vi "Single Slow IV v1.1.vi"() -> ()   [LabVIEW 2018]
uses:
  <vilib>/Utility/file.llb/Write Delimited Spreadsheet (DBL).vi
panel:
  in  "stop":bool
  in  "Tab Control 2":enum32{"Plot 0", "Plot 1", "Plot 2", "Plot 3"}(tab)
  out "I vs Chan 0":cluster{"Y":dbl[], "Y":dbl[]}[](graph)=[{"Y"=[-10.0, -9.9, -9.8, -9.7, -9.6, -9.5, -9.399999999999999, -9.299999999999999, -9.200000000000001, -9.1, -9.0, -8.9, -8.8, -8.7, -8.6, -8.5, -8.4, -8.299999999999999, -8.200000000000001, -8.100000000000001, -8.0, -7.9, -7.800000000000001, -7.7, -7.6, -7.5, -7.4, -7.3, -7.199999999999999, -7.1, -7.0, -6.8999999999999995, -6.799999999999999, -6.699999999999999, -6.6, -6.499999999999999, -6.4, -6.3, -6.2, -6.1, -6.0, -5.8999999999999995, -5.800000000000001, -5.700000000000001, -5.6000000000000005, -5.5, -5.4, -5.300000000000001, -5.2, -5.1, -5.0, -4.9, -4.8, -4.699999999999999, -4.6, -4.5, -4.3999999999999995, -4.299999999999999, -4.2, -4.1000000000000005, -4.0, -3.9000000000000004, -3.8, -3.7, -3.5999999999999996, -3.5, -3.3999999999999995, -3.3, -3.1999999999999993, -3.0999999999999996, -2.999999999999999, -2.9000000000000004, -2.8000000000000003, -2.7, -2.6, -2.5, -2.4, -2.3, -2.1999999999999997, -2.0999999999999996, -1.9999999999999996, -1.8999999999999995, -1.7999999999999994, -1.6999999999999993, -1.6000000000000003, -1.5000000000000002, -1.4000000000000001, -1.3, -1.2, -1.0999999999999999, -0.9999999999999998, -0.8999999999999997, -0.7999999999999996, -0.6999999999999995, -0.5999999999999994, -0.49999999999999933, -0.40000000000000036, -0.30000000000000027, -0.20000000000000018, -0.10000000000000009, 0.0, 0.10000000000000009, 0.20000000000000018, 0.30000000000000027, 0.40000000000000036, 0.5000000000000004, 0.6000000000000005, 0.7000000000000006, 0.8000000000000007, 0.9000000000000008, 1.0000000000000009, 1.100000000000001, 1.200000000000001, 1.3000000000000012, 1.4000000000000012, 1.5000000000000013, 1.5999999999999992, 1.6999999999999993, 1.7999999999999994, 1.8999999999999995, 1.9999999999999996, 2.0999999999999996, 2.1999999999999997, 2.3, 2.4, 2.5, 2.6, 2.7, 2.8000000000000003, 2.9000000000000004, 3.0000000000000004, 3.1000000000000005, 3.2000000000000006, 3.3000000000000007, 3.400000000000001, 3.500000000000001, 3.600000000000001, 3.700000000000001, 3.800000000000001, 3.9000000000000012, 4.000000000000002, 4.1, 4.199999999999999, 4.299999999999999, 4.3999999999999995, 4.5, 4.6, 4.699999999999999, 4.8, 4.9, 5.0, 5.1, 5.2, 5.300000000000001, 5.4, 5.5, 5.6000000000000005, 5.700000000000001, 5.800000000000001, 5.9, 6.000000000000001, 6.100000000000001, 6.200000000000001, 6.300000000000001, 6.400000000000001, 6.500000000000002, 6.600000000000001, 6.699999999999999, 6.799999999999999, 6.8999999999999995, 7.0, 7.1, 7.199999999999999, 7.3, 7.4, 7.5, 7.6, 7.7, 7.800000000000001, 7.9, 8.0, 8.100000000000001, 8.200000000000001, 8.3, 8.4, 8.5, 8.600000000000001, 8.700000000000001, 8.8, 8.900000000000002, 9.000000000000002, 9.100000000000001, 9.2, 9.299999999999999, 9.399999999999999, 9.5, 9.6, 9.7, 9.8, 9.9, 10.0], "Y"=[-0.00012308349609375, -0.0001234375, -0.00012093505859375, -0.00011771240234374999, -0.00011741943359375, -0.0001174072265625, -0.00011278076171874999, -0.00011287841796875001, -0.000112548828125, -0.00011116943359375001, -0.00010870361328125001, -0.00010834960937500001, -0.00010524902343750001, -0.00010374755859375, -0.00010172119140624999, -0.000101708984375, -0.00010029296875, -9.809570312500001e-05, -9.749755859375001e-05, -9.554443359375001e-05, -9.404296875e-05, -9.383544921875e-05, -9.218750000000001e-05, -8.903808593749999e-05, -8.939208984375e-05, -8.759765625e-05, -8.40087890625e-05, -8.4423828125e-05, -8.291015625e-05, -8.004150390625001e-05, -7.958984375e-05, -7.987060546875e-05, -7.769775390625001e-05, -7.576904296875e-05, -7.4658203125e-05, -7.2802734375e-05, -7.19482421875e-05, -7.186279296875001e-05, -6.826171875e-05, -6.763916015625e-05, -6.571044921875e-05, -6.614990234374999e-05, -6.256103515625e-05, -6.253662109375e-05, -5.97900390625e-05, -6.002197265625e-05, -5.882568359375e-05, -5.814208984375e-05, -5.416259765625e-05, -5.549316406250001e-05, -5.067138671875e-05, -5.35888671875e-05, -5.003662109375e-05, -4.7900390624999996e-05, -4.786376953125e-05, -4.3701171875e-05, -4.373779296875e-05, -4.140625e-05, -4.14306640625e-05, -3.7939453125e-05, -3.98193359375e-05, -3.8134765625e-05, -3.443603515625e-05, -3.5791015625e-05, -3.282470703125e-05, -3.2153320312499996e-05, -2.8991699218750002e-05, -2.92724609375e-05, -2.63916015625e-05, -2.52197265625e-05, -2.432861328125e-05, -2.05810546875e-05, -2.22412109375e-05, -2.122802734375e-05, -1.9128417968749997e-05, -1.689453125e-05, -1.826171875e-05, -1.612548828125e-05, -1.339111328125e-05, -1.2646484375e-05, -1.1462402343750001e-05, -9.99755859375e-06, -1.046142578125e-05, -8.5205078125e-06, -5.3466796875e-06, -4.101562500000001e-06, -5.944824218750001e-06, -2.099609375e-06, -1.2695312500000002e-06, 2.3193359375e-07, 3.18603515625e-06, 3.3691406250000004e-06, 6.4941406250000005e-06, 6.99462890625e-06, 6.99462890625e-06, 9.66796875e-06, 1.053466796875e-05, 1.2292480468750001e-05, 1.484375e-05, 1.5002441406250001e-05, 1.539306640625e-05, 1.497802734375e-05, 1.7041015625e-05, 2.073974609375e-05, 1.790771484375e-05, 1.9860839843749998e-05, 2.314453125e-05, 2.535400390625e-05, 2.801513671875e-05, 3.09814453125e-05, 2.987060546875e-05, 3.109130859375e-05, 3.3544921875000005e-05, 3.33984375e-05, 3.372802734375e-05, 3.5546875e-05, 3.8281250000000006e-05, 3.77685546875e-05, 3.85986328125e-05, 4.088134765625e-05, 4.32373046875e-05, 4.583740234375e-05, 4.6875e-05, 4.798583984375e-05, 4.942626953125e-05, 4.9621582031250003e-05, 4.8864746093750005e-05, 5.260009765625e-05, 5.27587890625e-05, 5.6555175781250006e-05, 5.62255859375e-05, 5.919189453125e-05, 5.92529296875e-05, 5.968017578125e-05, 6.07666015625e-05, 6.392822265625e-05, 6.356201171875e-05, 6.614990234374999e-05, 6.651611328124999e-05, 7.0654296875e-05, 6.744384765625e-05, 7.159423828125e-05, 7.252197265625001e-05, 7.586669921875e-05, 7.644042968750001e-05, 8.035888671875e-05, 7.917480468750001e-05, 8.00048828125e-05, 8.186035156250001e-05, 8.016357421875001e-05, 8.482666015625e-05, 8.565673828125001e-05, 8.717041015625001e-05, 8.928222656249999e-05, 8.980712890625e-05, 9.084472656250001e-05, 9.117431640625e-05, 9.261474609375e-05, 9.58251953125e-05, 9.794921875e-05, 9.8876953125e-05, 0.0001031494140625, 0.00010015869140625, 0.00010286865234375001, 0.00010465087890625, 0.00010682373046875, 0.00010622558593750001, 0.00011091308593750001, 0.00011068115234375001, 0.00010891113281250001, 0.000113916015625, 0.00011505126953125, 0.00011524658203125, 0.00011818847656250001, 0.00011900634765625, 0.00012003173828125, 0.00012119140625, 0.0001236083984375, 0.000122900390625, 0.0001267822265625, 0.00012701416015625, 0.00012807617187500002, 0.00013043212890625, 0.00013155517578125, 0.00013193359375, 0.00013393554687500002, 0.00013890380859375002, 0.00013798828125, 0.00013800048828125, 0.00014044189453125, 0.00014061279296875002, 0.000144677734375, 0.0001461181640625, 0.000145361328125, 0.00014764404296875, 0.00014439697265625, 0.00014951171874999999, 0.00014968261718750002, 0.00015272216796874999, 0.00015264892578125, 0.000153466796875]}]
  out "Name 0":string="DC Voltage V"
  out "I vs Chan 1":cluster{"Y":dbl[], "Y":dbl[]}[](graph)=[{"Y"=[-10.0, -9.9, -9.8, -9.7, -9.6, -9.5, -9.399999999999999, -9.299999999999999, -9.200000000000001, -9.1, -9.0, -8.9, -8.8, -8.7, -8.6, -8.5, -8.4, -8.299999999999999, -8.200000000000001, -8.100000000000001, -8.0, -7.9, -7.800000000000001, -7.7, -7.6, -7.5, -7.4, -7.3, -7.199999999999999, -7.1, -7.0, -6.8999999999999995, -6.799999999999999, -6.699999999999999, -6.6, -6.499999999999999, -6.4, -6.3, -6.2, -6.1, -6.0, -5.8999999999999995, -5.800000000000001, -5.700000000000001, -5.6000000000000005, -5.5, -5.4, -5.300000000000001, -5.2, -5.1, -5.0, -4.9, -4.8, -4.699999999999999, -4.6, -4.5, -4.3999999999999995, -4.299999999999999, -4.2, -4.1000000000000005, -4.0, -3.9000000000000004, -3.8, -3.7, -3.5999999999999996, -3.5, -3.3999999999999995, -3.3, -3.1999999999999993, -3.0999999999999996, -2.999999999999999, -2.9000000000000004, -2.8000000000000003, -2.7, -2.6, -2.5, -2.4, -2.3, -2.1999999999999997, -2.0999999999999996, -1.9999999999999996, -1.8999999999999995, -1.7999999999999994, -1.6999999999999993, -1.6000000000000003, -1.5000000000000002, -1.4000000000000001, -1.3, -1.2, -1.0999999999999999, -0.9999999999999998, -0.8999999999999997, -0.7999999999999996, -0.6999999999999995, -0.5999999999999994, -0.49999999999999933, -0.40000000000000036, -0.30000000000000027, -0.20000000000000018, -0.10000000000000009, 0.0, 0.10000000000000009, 0.20000000000000018, 0.30000000000000027, 0.40000000000000036, 0.5000000000000004, 0.6000000000000005, 0.7000000000000006, 0.8000000000000007, 0.9000000000000008, 1.0000000000000009, 1.100000000000001, 1.200000000000001, 1.3000000000000012, 1.4000000000000012, 1.5000000000000013, 1.5999999999999992, 1.6999999999999993, 1.7999999999999994, 1.8999999999999995, 1.9999999999999996, 2.0999999999999996, 2.1999999999999997, 2.3, 2.4, 2.5, 2.6, 2.7, 2.8000000000000003, 2.9000000000000004, 3.0000000000000004, 3.1000000000000005, 3.2000000000000006, 3.3000000000000007, 3.400000000000001, 3.500000000000001, 3.600000000000001, 3.700000000000001, 3.800000000000001, 3.9000000000000012, 4.000000000000002, 4.1, 4.199999999999999, 4.299999999999999, 4.3999999999999995, 4.5, 4.6, 4.699999999999999, 4.8, 4.9, 5.0, 5.1, 5.2, 5.300000000000001, 5.4, 5.5, 5.6000000000000005, 5.700000000000001, 5.800000000000001, 5.9, 6.000000000000001, 6.100000000000001, 6.200000000000001, 6.300000000000001, 6.400000000000001, 6.500000000000002, 6.600000000000001, 6.699999999999999, 6.799999999999999, 6.8999999999999995, 7.0, 7.1, 7.199999999999999, 7.3, 7.4, 7.5, 7.6, 7.7, 7.800000000000001, 7.9, 8.0, 8.100000000000001, 8.200000000000001, 8.3, 8.4, 8.5, 8.600000000000001, 8.700000000000001, 8.8, 8.900000000000002, 9.000000000000002, 9.100000000000001, 9.2, 9.299999999999999, 9.399999999999999, 9.5, 9.6, 9.7, 9.8, 9.9, 10.0], "Y"=[-9.593505859375, -9.5345458984375, -9.409423828125, -9.3255615234375, -9.232177734375, -9.154541015625, -9.0064697265625, -8.9058837890625, -8.836181640625, -8.7589111328125, -8.6331787109375, -8.5640869140625, -8.447265625, -8.3675537109375, -8.2216796875, -8.175537109375, -8.065185546875, -7.9620361328125, -7.8717041015625, -7.77880859375, -7.6875, -7.6253662109375, -7.516357421875, -7.3792724609375, -7.2818603515625, -7.2069091796875, -7.0982666015625, -7.0257568359375, -6.923583984375, -6.798583984375, -6.7196044921875, -6.6395263671875, -6.5299072265625, -6.4405517578125, -6.3487548828125, -6.248046875, -6.1641845703125, -6.0799560546875, -5.965087890625, -5.882080078125, -5.7880859375, -5.7003173828125, -5.58544921875, -5.485595703125, -5.3775634765625, -5.3094482421875, -5.2239990234375, -5.120361328125, -4.9964599609375, -4.9444580078125, -4.79248046875, -4.744873046875, -4.6241455078125, -4.5133056640625, -4.4425048828125, -4.3153076171875, -4.248046875, -4.1307373046875, -4.0538330078125, -3.9373779296875, -3.8994140625, -3.782470703125, -3.6390380859375, -3.598388671875, -3.4920654296875, -3.395751953125, -3.2786865234375, -3.2120361328125, -3.0963134765625, -3.002197265625, -2.9107666015625, -2.75732421875, -2.713623046875, -2.621826171875, -2.535888671875, -2.4136962890625, -2.372802734375, -2.2467041015625, -2.124267578125, -2.048095703125, -1.9478759765625, -1.8392333984375, -1.8209228515625, -1.7073974609375, -1.562255859375, -1.4957275390625, -1.4473876953125, -1.306640625, -1.2362060546875, -1.1260986328125, -0.9921875, -0.931640625, -0.8140869140625, -0.73583984375, -0.6666259765625, -0.527587890625, -0.4603271484375, -0.361083984375, -0.2269287109375, -0.1763916015625, -0.08984375, 0.015380859375, 0.1270751953125, 0.263427734375, 0.3182373046875, 0.38037109375, 0.48974609375, 0.59765625, 0.70166015625, 0.8580322265625, 0.88330078125, 0.9742431640625, 1.094482421875, 1.1697998046875, 1.2156982421875, 1.35595703125, 1.4716796875, 1.5325927734375, 1.6243896484375, 1.7108154296875, 1.84130859375, 1.951171875, 2.045654296875, 2.146728515625, 2.2236328125, 2.3109130859375, 2.37353515625, 2.49951171875, 2.59033203125, 2.6856689453125, 2.7845458984375, 2.8961181640625, 2.9559326171875, 3.0474853515625, 3.1373291015625, 3.2685546875, 3.3409423828125, 3.439697265625, 3.530029296875, 3.6690673828125, 3.70556640625, 3.832275390625, 3.9168701171875, 4.0284423828125, 4.1300048828125, 4.2607421875, 4.3009033203125, 4.4122314453125, 4.49609375, 4.56201171875, 4.6815185546875, 4.7872314453125, 4.8818359375, 4.9942626953125, 5.055419921875, 5.160888671875, 5.231689453125, 5.3519287109375, 5.4739990234375, 5.56298828125, 5.6533203125, 5.7923583984375, 5.806396484375, 5.936767578125, 6.0274658203125, 6.14111328125, 6.2001953125, 6.37353515625, 6.431640625, 6.496826171875, 6.6165771484375, 6.7174072265625, 6.79345703125, 6.9200439453125, 6.97900390625, 7.0965576171875, 7.176025390625, 7.3065185546875, 7.365966796875, 7.5006103515625, 7.5654296875, 7.6612548828125, 7.7730712890625, 7.868408203125, 7.9364013671875, 8.0616455078125, 8.1871337890625, 8.2489013671875, 8.3131103515625, 8.435791015625, 8.5284423828125, 8.630126953125, 8.75, 8.8126220703125, 8.908203125, 8.9510498046875, 9.1063232421875, 9.17236328125, 9.272705078125, 9.370361328125, 9.4595947265625]}]
  out "Name 1":string="DC current uA"
  out "I vs Chan 2":cluster{"Y":dbl[], "Y":dbl[]}[](graph)=[{"Y"=[-10.0, -9.9, -9.8, -9.7, -9.6, -9.5, -9.399999999999999, -9.299999999999999, -9.200000000000001, -9.1, -9.0, -8.9, -8.8, -8.7, -8.6, -8.5, -8.4, -8.299999999999999, -8.200000000000001, -8.100000000000001, -8.0, -7.9, -7.800000000000001, -7.7, -7.6, -7.5, -7.4, -7.3, -7.199999999999999, -7.1, -7.0, -6.8999999999999995, -6.799999999999999, -6.699999999999999, -6.6, -6.499999999999999, -6.4, -6.3, -6.2, -6.1, -6.0, -5.8999999999999995, -5.800000000000001, -5.700000000000001, -5.6000000000000005, -5.5, -5.4, -5.300000000000001, -5.2, -5.1, -5.0, -4.9, -4.8, -4.699999999999999, -4.6, -4.5, -4.3999999999999995, -4.299999999999999, -4.2, -4.1000000000000005, -4.0, -3.9000000000000004, -3.8, -3.7, -3.5999999999999996, -3.5, -3.3999999999999995, -3.3, -3.1999999999999993, -3.0999999999999996, -2.999999999999999, -2.9000000000000004, -2.8000000000000003, -2.7, -2.6, -2.5, -2.4, -2.3, -2.1999999999999997, -2.0999999999999996, -1.9999999999999996, -1.8999999999999995, -1.7999999999999994, -1.6999999999999993, -1.6000000000000003, -1.5000000000000002, -1.4000000000000001, -1.3, -1.2, -1.0999999999999999, -0.9999999999999998, -0.8999999999999997, -0.7999999999999996, -0.6999999999999995, -0.5999999999999994, -0.49999999999999933, -0.40000000000000036, -0.30000000000000027, -0.20000000000000018, -0.10000000000000009, 0.0, 0.10000000000000009, 0.20000000000000018, 0.30000000000000027, 0.40000000000000036, 0.5000000000000004, 0.6000000000000005, 0.7000000000000006, 0.8000000000000007, 0.9000000000000008, 1.0000000000000009, 1.100000000000001, 1.200000000000001, 1.3000000000000012, 1.4000000000000012, 1.5000000000000013, 1.5999999999999992, 1.6999999999999993, 1.7999999999999994, 1.8999999999999995, 1.9999999999999996, 2.0999999999999996, 2.1999999999999997, 2.3, 2.4, 2.5, 2.6, 2.7, 2.8000000000000003, 2.9000000000000004, 3.0000000000000004, 3.1000000000000005, 3.2000000000000006, 3.3000000000000007, 3.400000000000001, 3.500000000000001, 3.600000000000001, 3.700000000000001, 3.800000000000001, 3.9000000000000012, 4.000000000000002, 4.1, 4.199999999999999, 4.299999999999999, 4.3999999999999995, 4.5, 4.6, 4.699999999999999, 4.8, 4.9, 5.0, 5.1, 5.2, 5.300000000000001, 5.4, 5.5, 5.6000000000000005, 5.700000000000001, 5.800000000000001, 5.9, 6.000000000000001, 6.100000000000001, 6.200000000000001, 6.300000000000001, 6.400000000000001, 6.500000000000002, 6.600000000000001, 6.699999999999999, 6.799999999999999, 6.8999999999999995, 7.0, 7.1, 7.199999999999999, 7.3, 7.4, 7.5, 7.6, 7.7, 7.800000000000001, 7.9, 8.0, 8.100000000000001, 8.200000000000001, 8.3, 8.4, 8.5, 8.600000000000001, 8.700000000000001, 8.8, 8.900000000000002, 9.000000000000002, 9.100000000000001, 9.2, 9.299999999999999, 9.399999999999999, 9.5, 9.6, 9.7, 9.8, 9.9, 10.0], "Y"=[0.14237060546875, 0.14224853515625, 0.13931884765625, 0.13436279296875, 0.13089599609375, 0.1484130859375, 0.1311767578125, 0.12135009765625, 0.126171875, 0.11885986328125, 0.12998046875, 0.1361572265625, 0.137744140625, 0.13939208984375, 0.14383544921875, 0.13359375, 0.1277099609375, 0.13414306640625, 0.1346923828125, 0.13975830078125, 0.12977294921875, 0.1345458984375, 0.13109130859375, 0.14085693359375, 0.1389892578125, 0.12850341796875, 0.132080078125, 0.1217529296875, 0.119287109375, 0.121826171875, 0.13089599609375, 0.13604736328125, 0.13546142578125, 0.12481689453125, 0.133984375, 0.14044189453125, 0.143896484375, 0.138916015625, 0.1323486328125, 0.1269287109375, 0.1247314453125, 0.13338623046875, 0.1311767578125, 0.1350341796875, 0.1343505859375, 0.1373291015625, 0.1375244140625, 0.14576416015625, 0.14306640625, 0.143408203125, 0.1353759765625, 0.1471435546875, 0.139111328125, 0.13782958984375, 0.14586181640625, 0.14405517578125, 0.12735595703125, 0.12763671875, 0.14405517578125, 0.1427734375, 0.131298828125, 0.135302734375, 0.134326171875, 0.13094482421875, 0.12060546875, 0.12052001953125, 0.12391357421875, 0.13721923828125, 0.13489990234375, 0.1359619140625, 0.1348388671875, 0.13406982421875, 0.1313232421875, 0.1314453125, 0.13187255859375, 0.128076171875, 0.12703857421875, 0.135888671875, 0.12996826171875, 0.1257080078125, 0.1363037109375, 0.12720947265625, 0.124462890625, 0.13179931640625, 0.13096923828125, 0.13603515625, 0.13265380859375, 0.1372314453125, 0.14005126953125, 0.13939208984375, 0.1390380859375, 0.14755859375, 0.14853515625, 0.15540771484375, 0.14439697265625, 0.15701904296875, 0.15970458984375, 0.14603271484375, 0.11851806640625, 0.08155517578125, 0.0737548828125, 0.059033203125, 0.0862548828125, 0.107373046875, 0.14686279296875, 0.153271484375, 0.16593017578125, 0.16634521484375, 0.15345458984375, 0.154052734375, 0.14573974609375, 0.13909912109375, 0.1457275390625, 0.144091796875, 0.13836669921875, 0.12183837890625, 0.12923583984375, 0.13216552734375, 0.13109130859375, 0.12672119140625, 0.12862548828125, 0.138720703125, 0.13399658203125, 0.13165283203125, 0.14306640625, 0.131005859375, 0.12864990234375, 0.124072265625, 0.13448486328125, 0.1269775390625, 0.13427734375, 0.12752685546875, 0.1389892578125, 0.1315185546875, 0.11864013671875, 0.119140625, 0.12742919921875, 0.13262939453125, 0.13258056640625, 0.13468017578125, 0.139892578125, 0.1356201171875, 0.1286865234375, 0.11729736328125, 0.12257080078125, 0.11641845703125, 0.137060546875, 0.14832763671875, 0.1409423828125, 0.13443603515625, 0.1446044921875, 0.13297119140625, 0.13448486328125, 0.1262451171875, 0.127734375, 0.131103515625, 0.14002685546875, 0.12392578125, 0.12786865234375, 0.11773681640625, 0.12716064453125, 0.12587890625, 0.1200439453125, 0.13533935546875, 0.12574462890625, 0.1306640625, 0.14171142578125, 0.1371826171875, 0.13031005859375, 0.1381591796875, 0.12945556640625, 0.13642578125, 0.14312744140625, 0.13961181640625, 0.14447021484375, 0.13270263671875, 0.1308349609375, 0.136376953125, 0.1431396484375, 0.13074951171875, 0.12476806640625, 0.1382568359375, 0.1403076171875, 0.1392578125, 0.12987060546875, 0.13812255859375, 0.14114990234375, 0.142626953125, 0.1402587890625, 0.14439697265625, 0.145849609375, 0.14061279296875, 0.12906494140625, 0.1228759765625, 0.12764892578125, 0.130908203125, 0.134765625, 0.1360107421875, 0.13594970703125, 0.13138427734375, 0.134765625]}]
  out "Name 2":string="dV V"
  out "I vs Chan 3":cluster{"Y":dbl[], "Y":dbl[]}[](graph)=[{"Y"=[-10.0, -9.9, -9.8, -9.7, -9.6, -9.5, -9.399999999999999, -9.299999999999999, -9.200000000000001, -9.1, -9.0, -8.9, -8.8, -8.7, -8.6, -8.5, -8.4, -8.299999999999999, -8.200000000000001, -8.100000000000001, -8.0, -7.9, -7.800000000000001, -7.7, -7.6, -7.5, -7.4, -7.3, -7.199999999999999, -7.1, -7.0, -6.8999999999999995, -6.799999999999999, -6.699999999999999, -6.6, -6.499999999999999, -6.4, -6.3, -6.2, -6.1, -6.0, -5.8999999999999995, -5.800000000000001, -5.700000000000001, -5.6000000000000005, -5.5, -5.4, -5.300000000000001, -5.2, -5.1, -5.0, -4.9, -4.8, -4.699999999999999, -4.6, -4.5, -4.3999999999999995, -4.299999999999999, -4.2, -4.1000000000000005, -4.0, -3.9000000000000004, -3.8, -3.7, -3.5999999999999996, -3.5, -3.3999999999999995, -3.3, -3.1999999999999993, -3.0999999999999996, -2.999999999999999, -2.9000000000000004, -2.8000000000000003, -2.7, -2.6, -2.5, -2.4, -2.3, -2.1999999999999997, -2.0999999999999996, -1.9999999999999996, -1.8999999999999995, -1.7999999999999994, -1.6999999999999993, -1.6000000000000003, -1.5000000000000002, -1.4000000000000001, -1.3, -1.2, -1.0999999999999999, -0.9999999999999998, -0.8999999999999997, -0.7999999999999996, -0.6999999999999995, -0.5999999999999994, -0.49999999999999933, -0.40000000000000036, -0.30000000000000027, -0.20000000000000018, -0.10000000000000009, 0.0, 0.10000000000000009, 0.20000000000000018, 0.30000000000000027, 0.40000000000000036, 0.5000000000000004, 0.6000000000000005, 0.7000000000000006, 0.8000000000000007, 0.9000000000000008, 1.0000000000000009, 1.100000000000001, 1.200000000000001, 1.3000000000000012, 1.4000000000000012, 1.5000000000000013, 1.5999999999999992, 1.6999999999999993, 1.7999999999999994, 1.8999999999999995, 1.9999999999999996, 2.0999999999999996, 2.1999999999999997, 2.3, 2.4, 2.5, 2.6, 2.7, 2.8000000000000003, 2.9000000000000004, 3.0000000000000004, 3.1000000000000005, 3.2000000000000006, 3.3000000000000007, 3.400000000000001, 3.500000000000001, 3.600000000000001, 3.700000000000001, 3.800000000000001, 3.9000000000000012, 4.000000000000002, 4.1, 4.199999999999999, 4.299999999999999, 4.3999999999999995, 4.5, 4.6, 4.699999999999999, 4.8, 4.9, 5.0, 5.1, 5.2, 5.300000000000001, 5.4, 5.5, 5.6000000000000005, 5.700000000000001, 5.800000000000001, 5.9, 6.000000000000001, 6.100000000000001, 6.200000000000001, 6.300000000000001, 6.400000000000001, 6.500000000000002, 6.600000000000001, 6.699999999999999, 6.799999999999999, 6.8999999999999995, 7.0, 7.1, 7.199999999999999, 7.3, 7.4, 7.5, 7.6, 7.7, 7.800000000000001, 7.9, 8.0, 8.100000000000001, 8.200000000000001, 8.3, 8.4, 8.5, 8.600000000000001, 8.700000000000001, 8.8, 8.900000000000002, 9.000000000000002, 9.100000000000001, 9.2, 9.299999999999999, 9.399999999999999, 9.5, 9.6, 9.7, 9.8, 9.9, 10.0], "Y"=[0.94891357421875, 0.9578369140625, 0.94735107421875, 0.9477783203125, 0.94619140625, 0.95455322265625, 0.95579833984375, 0.94427490234375, 0.9491455078125, 0.9447021484375, 0.94097900390625, 0.9394775390625, 0.95335693359375, 0.9498779296875, 0.94693603515625, 0.9442138671875, 0.949609375, 0.947998046875, 0.952978515625, 0.9468017578125, 0.95482177734375, 0.9583984375, 0.947021484375, 0.94285888671875, 0.9375, 0.940478515625, 0.9356689453125, 0.94532470703125, 0.9408447265625, 0.93841552734375, 0.94471435546875, 0.93890380859375, 0.95328369140625, 0.93822021484375, 0.9506591796875, 0.94007568359375, 0.950927734375, 0.9435546875, 0.95013427734375, 0.9459716796875, 0.950537109375, 0.95440673828125, 0.95286865234375, 0.9526611328125, 0.95450439453125, 0.95272216796875, 0.95611572265625, 0.950537109375, 0.955322265625, 0.9569091796875, 0.957177734375, 0.93946533203125, 0.95079345703125, 0.952880859375, 0.9504150390625, 0.9560302734375, 0.94222412109375, 0.9494140625, 0.956005859375, 0.9582275390625, 0.95799560546875, 0.94637451171875, 0.9373046875, 0.94144287109375, 0.95390625, 0.94190673828125, 0.9397216796875, 0.9546142578125, 0.94547119140625, 0.9369384765625, 0.95045166015625, 0.94356689453125, 0.942578125, 0.94906005859375, 0.9567626953125, 0.943408203125, 0.94183349609375, 0.95521240234375, 0.9445068359375, 0.95048828125, 0.9523681640625, 0.95489501953125, 0.95279541015625, 0.9577880859375, 0.95416259765625, 0.95416259765625, 0.9467529296875, 0.94588623046875, 0.94029541015625, 0.9417236328125, 0.954345703125, 0.954736328125, 0.94490966796875, 0.94364013671875, 0.93758544921875, 0.95206298828125, 0.954296875, 0.94566650390625, 0.9493408203125, 0.95355224609375, 0.9425537109375, 0.94534912109375, 0.9372314453125, 0.93629150390625, 0.93914794921875, 0.9525146484375, 0.94290771484375, 0.94998779296875, 0.95157470703125, 0.94967041015625, 0.94981689453125, 0.94427490234375, 0.95389404296875, 0.94150390625, 0.94864501953125, 0.94586181640625, 0.951708984375, 0.9447021484375, 0.94300537109375, 0.9546142578125, 0.95369873046875, 0.95408935546875, 0.94371337890625, 0.945654296875, 0.9428466796875, 0.95032958984375, 0.946044921875, 0.95467529296875, 0.9572998046875, 0.94462890625, 0.95084228515625, 0.949560546875, 0.94622802734375, 0.94490966796875, 0.94464111328125, 0.94300537109375, 0.94691162109375, 0.94111328125, 0.93807373046875, 0.94560546875, 0.946630859375, 0.9541015625, 0.9412353515625, 0.9434814453125, 0.95244140625, 0.95382080078125, 0.955419921875, 0.95010986328125, 0.94884033203125, 0.9486572265625, 0.94893798828125, 0.94495849609375, 0.9525146484375, 0.95382080078125, 0.9568359375, 0.944921875, 0.95164794921875, 0.9466064453125, 0.9466552734375, 0.94083251953125, 0.93809814453125, 0.93897705078125, 0.94224853515625, 0.9445068359375, 0.94974365234375, 0.9420166015625, 0.94814453125, 0.9400634765625, 0.9485107421875, 0.94620361328125, 0.947998046875, 0.94503173828125, 0.941162109375, 0.94833984375, 0.9508544921875, 0.9482177734375, 0.9396240234375, 0.9502685546875, 0.95997314453125, 0.96004638671875, 0.9498779296875, 0.94691162109375, 0.95335693359375, 0.95001220703125, 0.94827880859375, 0.943408203125, 0.9549560546875, 0.9496826171875, 0.9443603515625, 0.94561767578125, 0.94581298828125, 0.9424072265625, 0.95430908203125, 0.94036865234375, 0.9526611328125, 0.9468017578125, 0.954443359375, 0.94600830078125, 0.94906005859375, 0.9413330078125, 0.93865966796875]}]
  out "Name 3":string="dI uA"
  in  "Tab Control":T1(tab)
  in  "cRIO IP":string="//172.22.11.2"
  in  "Reading Average times":i32=20
  out "Unit":string
  in  "Tab Control 3":enum32{"Current", "Magnetic field"}(tab)
  in  "Delay Time s":dbl=0.15 caption="Delay Time (s)"
  in  "AO Channel":string(combo)="AO0"
  in  "current output Scale factor":dbl=10.0
  in  "Device Select":string(combo)="Elsa Magnet"
  in  "Fixed current uA":dbl
  in  "Scale factor":dbl
  in  "Field Rate mT per sec":dbl=0.1 format="%#_13g"
  in  "Start":dbl=-10.0
  in  "Current Range":dbl=20.0
  in  "Current Step":dbl=0.1
  in  "Ramp type":string(combo)="Range"
  in  "Ramp up first T":bool=TRUE
  in  "Channel name 0":string(combo)="DC Voltage V"
  in  "Scale factor0":dbl=0.001
  in  "Scale factor1":dbl=10.0
  in  "Channel name 1":string(combo)="DC current uA"
  in  "Chan 1":bool=TRUE
  in  "Scale factor2":dbl=1.0
  in  "Channel name 2":string(combo)="dV V"
  in  "Chan 2":bool=TRUE
  in  "Scale factor3":dbl=1.0
  in  "Channel name 3":string(combo)="dI uA"
  in  "Chan 3":bool=TRUE
  in  "Contour plot folder":path=path "C:/Users/gyue/Box/Guang Yue uiuc research box folder/data"
  out "error out":errorcluster
  # "Voltage x factor=uA"
  # "Voltage x factor=uA"
  # "Voltage x factor=actual"
  # "Voltage x factor=actual"
  # "Voltage x factor=actual"
  # "Voltage x factor=actual"
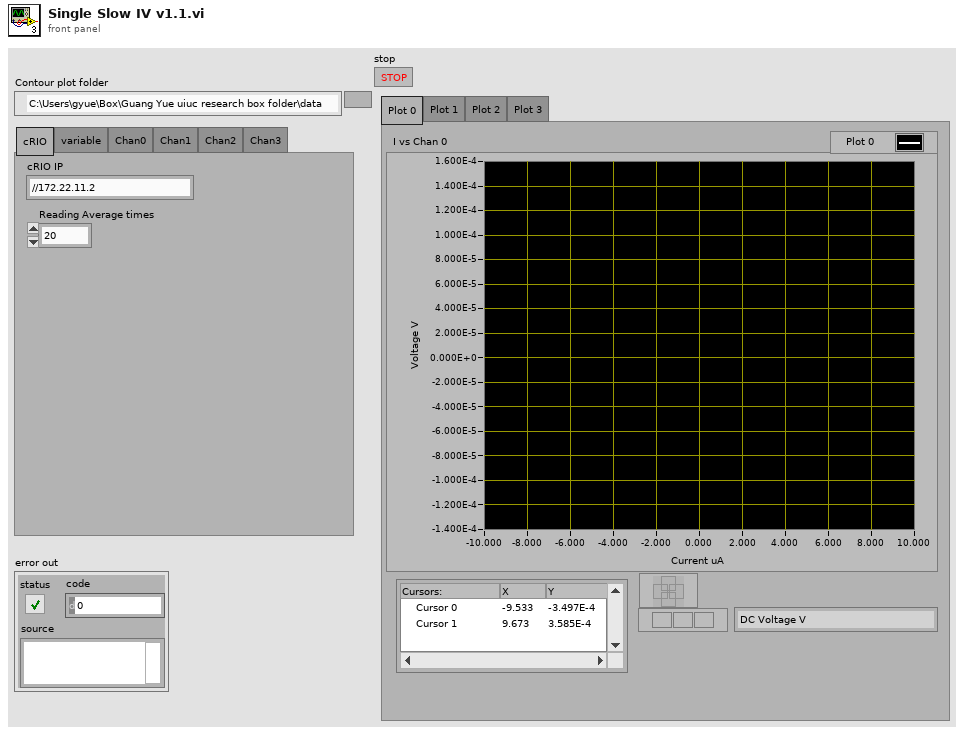
[diagram p1: front panel]
types:
  T1 = enum32{"cRIO", "variable", "Chan0", "Chan1", "Chan2", "Chan3"}
  T2 = cluster{"AI0":dbl, "AI1":dbl, "AI2":dbl, "AI3":dbl}
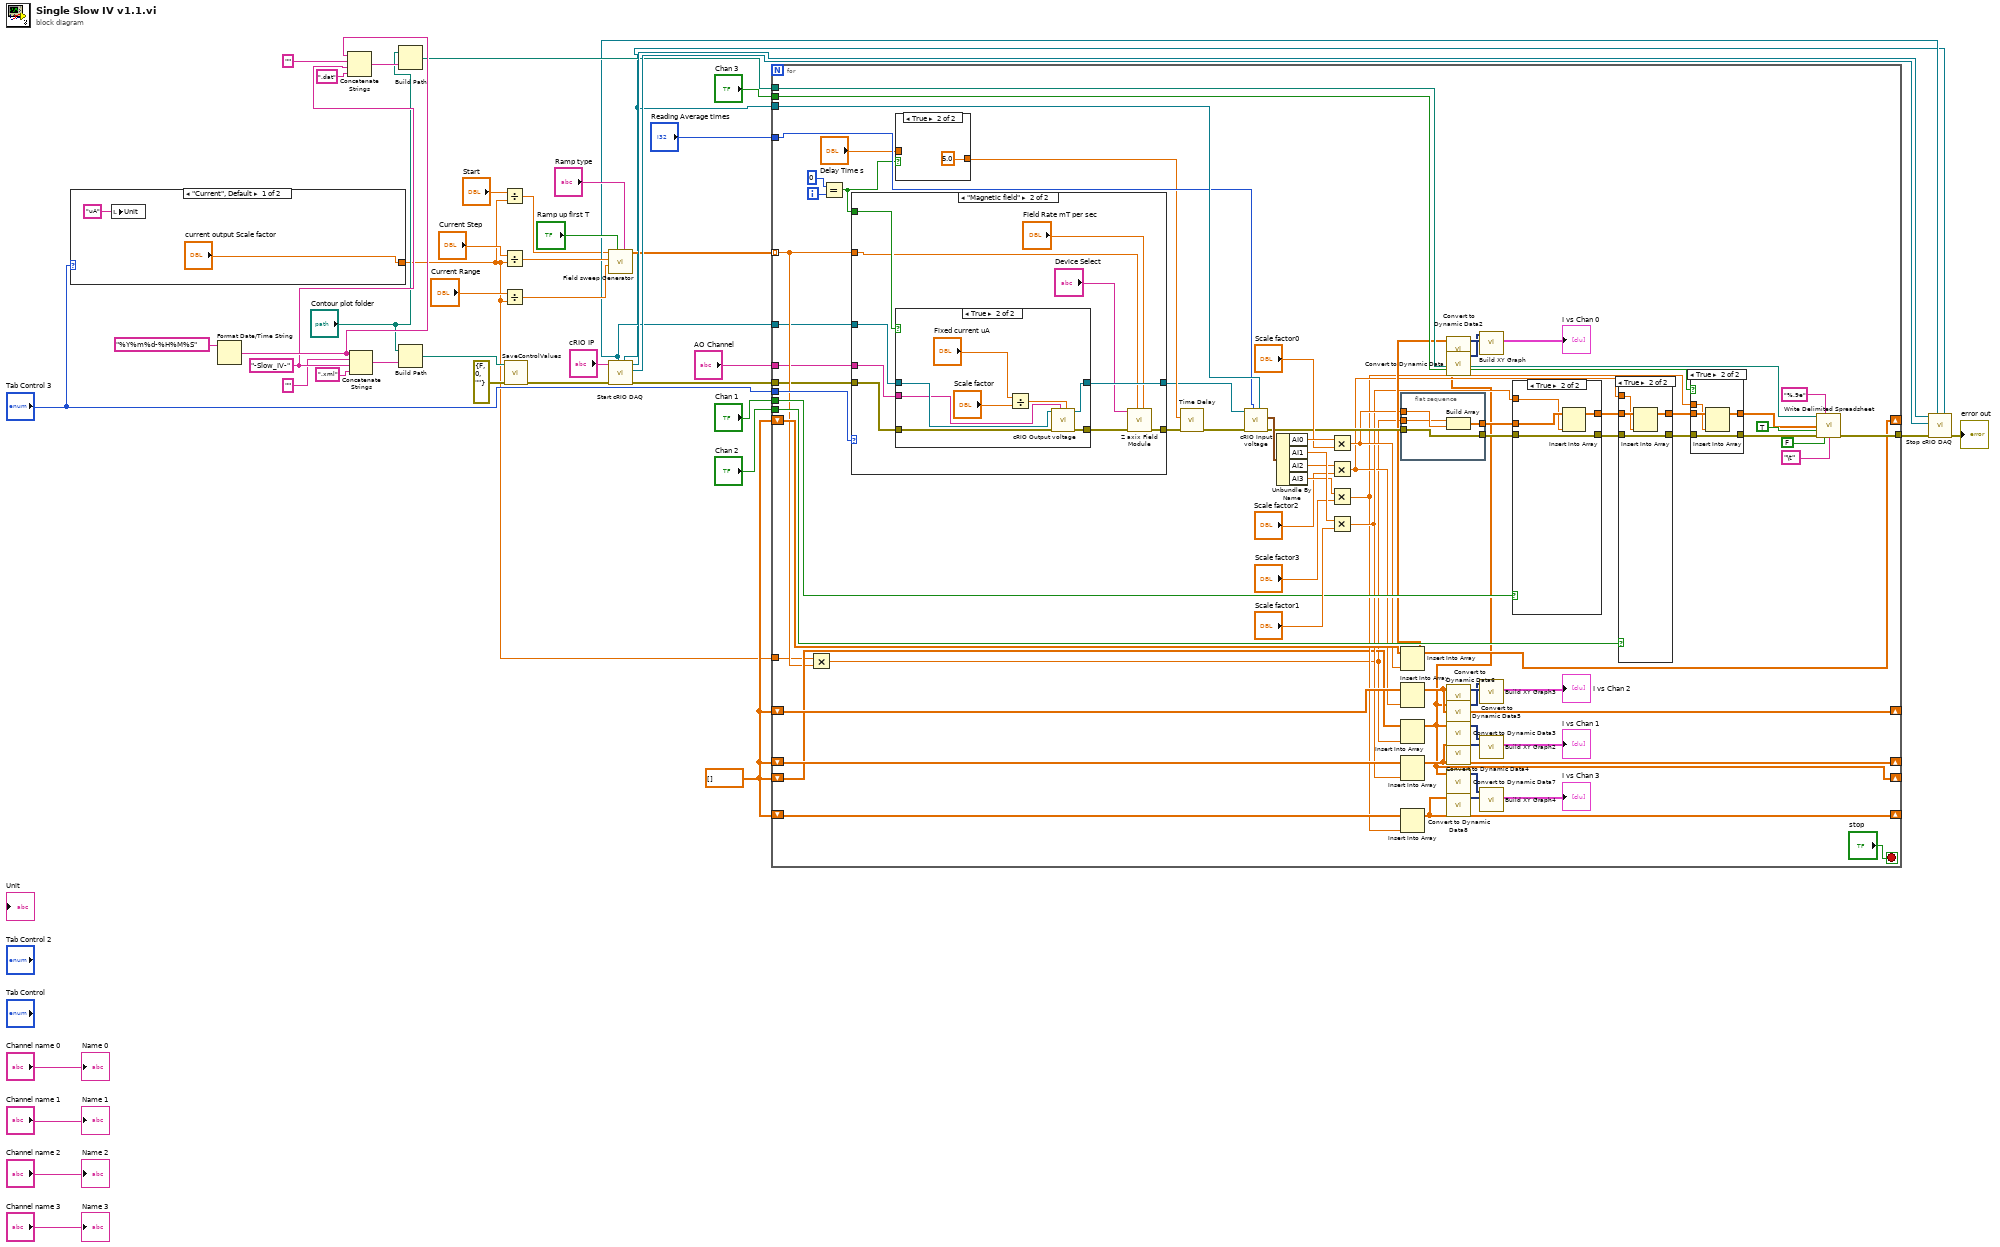
[diagram p0: block diagram]
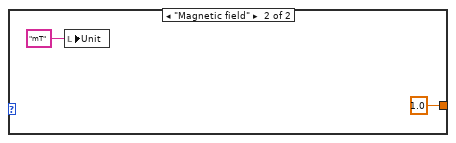
[diagram p2: hidden frame]
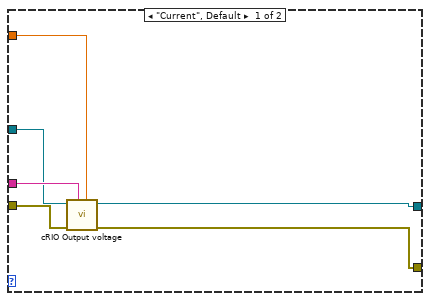
[diagram p3: hidden frame]
diagram:
  w11 = dbl[] []
  w36 = "-Slow_IV-"
  n1 = case shown="\"Current\", Default" "Tab Control 3" {
    tunnel: ["current output Scale factor" 1.0 ("current output Scale factor")] -> w1
    frame "Current", Default {
      n2 = local write "Unit"("uA" ("Unit")) -> ()
    }
    frame "Magnetic field" {
      n3 = local write "Unit"("mT" ("Unit")) -> ()
    }
  }
  n4 = Format Date/Time String(time format string (%c)="%Y%m%d-%H%M%S") -> (date/time string=w37:string)  [unwired: 2 in]
  n5 = Concatenate Strings(w37, "" ("string"), w36, ".dat" ("string")) -> (w39:string)
  n6 = Concatenate Strings(w37, "" ("string"), w36, ".xml" ("string")) -> (w42:string)
  n7 = Build Path(base path="Contour plot folder", name or relative path=w39) -> (appended path=w19:path)
  n8 = Build Path(base path="Contour plot folder", name or relative path=w42) -> (appended path=w40:path)
  n9 = Divide(x="Start", y=w1) -> (x/y=w3:dbl)
  n10 = Divide(x="Current Step", y=w1) -> (x/y=w24:dbl)
  n11 = Divide(x="Current Range", y=w1) -> (x/y=w23:dbl)
  n12 = call "SaveControlValues.vi"("XML File Path"=w40, "error in (no error)"=errorcluster {"status"=FALSE, "code"=0, "source"=""} ("error in")) -> ("error out"=w33:errorcluster)  [unwired: 8 in]
  n13 = call "Field sweep Generator.vi"("Ramp type"="Ramp type", "Ramp up first T"="Ramp up first T", "Field Radius"=w23, "Field step"=w24, "Field Origin"=w3) -> ("output array"=w20:dbl[])  [unwired: 6 in]
  n14 = call "Start cRIO DAQ.vi"("error in (no error)"=w33, "cRIO IP"="cRIO IP") -> ("error out"=w22:errorcluster, "vi reference"=w31:refnum<vi>, "application reference"=w32:refnum<vi>, "DAQ_AI_Reader endpoint"=w17:refnum<k21>, "DAQ_CMD_Writer endpoint"=w18:refnum<k21>)  [unwired: 5 in]
  n15 = for {
    tunnel: w22 -> [w53]
    tunnel: w18 -> [w52]
    tunnel: "AO Channel" -> [w54]
    tunnel: w20 -> [w55] mode=indexing
    tunnel: w17 -> [w118]
    tunnel: w19 -> [w117]
    tunnel: "Chan 1" -> [w99]
    tunnel: "Chan 2" -> [w98]
    tunnel: "Chan 3" -> [w97]
    tunnel: [w78] -> w10
    shift-right: [w73] -> _
    shift-left: w11 -> [w77]
    shift-right: [w72] -> _
    shift-left: w11 -> [w76]
    shift-right: [w71] -> _
    shift-left: w11 -> [w75]
    shift-right: [w70] -> _
    shift-left: w11 -> [w74]
    shift-right: [w63] -> _
    shift-left: w11 -> [w65]
    tunnel: "Reading Average times" -> [w62]
    tunnel: "Tab Control 3" -> [w56]
    tunnel: w1 -> [w48]
    i -> [w60]
    stop <- "stop" stop-if-true
    n16 = Multiply(x=w48, y=w55) -> (x*y=w64:dbl)
    n17 = Equal?(x=0, y=w60) -> (x = y?=w49:bool)
    n18 = case shown="\"Magnetic field\"" w56 {
      tunnel: w55 -> [w124 w125]
      tunnel: w54 -> [w123 w130]
      tunnel: w53 -> [w122 w133]
      tunnel: w52 -> [w121 w132]
      tunnel: [w120 w128] -> w51
      tunnel: [w119 w131] -> w50
      tunnel: w49 -> [_ w134]
      frame "Current", Default {
        n19 = call "cRIO Output voltage.vi"("Voltage"=w124, "AO Channel"=w123, "error in (no error)"=w122, "DAQ_CMD_Writer endpoint"=w121) -> ("error out"=w120:errorcluster, "DAQ_CMD_Writer endpoint out"=w119:refnum<k21>)  [unwired: 6 in]
      }
      frame "Magnetic field" {
        n20 = case shown="True" w134 {
          tunnel: w133 -> [w135 w144]
          tunnel: [w135 w143] -> w129
          tunnel: w132 -> [w136 w142]
          tunnel: [w136 w141] -> w131
          tunnel: w130 -> [_ w140]
          frame False {
          }
          frame True {
            n21 = Divide(x="Fixed current uA", y="Scale factor") -> (x/y=w138:dbl)
            n22 = call "cRIO Output voltage.vi"("Voltage"=w138, "AO Channel"=w140, "error in (no error)"=w144, "DAQ_CMD_Writer endpoint"=w142) -> ("error out"=w143:errorcluster, "DAQ_CMD_Writer endpoint out"=w141:refnum<k21>)  [unwired: 6 in]
          }
        }
        n23 = call "Z axix Field Module.vi"("Field Rate mT per sec"="Field Rate mT per sec", "Field Target mT"=w125, "error in (no error)"=w129, "Device Select"="Device Select") -> ("error out"=w128:errorcluster)  [unwired: 7 in]
      }
    }
    n24 = case shown="True" w49 {
      tunnel: "Delay Time s" -> [w145 _]
      tunnel: [w145 5.0 ("Delay Time s")] -> w57
      frame False {
      }
      frame True {
      }
    }
    n25 = call "Time Delay"("error in (no error)"=w51, "Delay Time (s)"=w57) -> ("error out"=w110:errorcluster)  [unwired: 9 in]
    n26 = call "cRIO Input voltage.vi"("DAQ_AI_Reader endpoint"=w118, "Average"=w62, "error in (no error)"=w110, "DAQ_CMD_Writer endpoint"=w50) -> ("error out"=w94:errorcluster, "output cluster"=w109:T2)  [unwired: 5 in, 1 out]
    n27 = Unbundle By Name(w109) -> ("AI0"=w108:dbl, "AI1"=w107:dbl, "AI2"=w106:dbl, "AI3"=w105:dbl)
    n28 = Multiply(x=w108, y="Scale factor0") -> (x*y=w69:dbl)
    n29 = Multiply(x=w106, y="Scale factor2") -> (x*y=w67:dbl)
    n30 = Multiply(x=w105, y="Scale factor3") -> (x*y=w66:dbl)
    n31 = Multiply(x=w107, y="Scale factor1") -> (x*y=w68:dbl)
    n32 = flat-sequence {
      tunnel: w94 -> [w150]
      tunnel: [w150] -> w93
      tunnel: w69 -> [w148]
      tunnel: [w149] -> w92
      tunnel: w64 -> [w147]
      frame #0 {
        n33 = Build Array(w147, w148) -> (w149:dbl[])
      }
    }
    n34 = Insert Into Array(array=w77, new element=w69) -> (w73:dbl[])  [unwired: 1 in]
    n35 = Insert Into Array(array=w75, new element=w67) -> (w71:dbl[])  [unwired: 1 in]
    n36 = Insert Into Array(array=w65, new element=w64) -> (w63:dbl[])  [unwired: 1 in]
    n37 = Insert Into Array(array=w76, new element=w68) -> (w72:dbl[])  [unwired: 1 in]
    n38 = Insert Into Array(array=w74, new element=w66) -> (w70:dbl[])  [unwired: 1 in]
    n39 = call "Convert to Dynamic Data2"("Array"=w73) -> ("Dynamic Data Type"=w113:dynamicdata)  [unwired: 3 in]
    n40 = call "Convert to Dynamic Data"("Array"=w63) -> ("Dynamic Data Type"=w112:dynamicdata)  [unwired: 3 in]
    n41 = call "Convert to Dynamic Data6"("Array"=w71) -> ("Dynamic Data Type"=w84:dynamicdata)  [unwired: 3 in]
    n42 = call "Convert to Dynamic Data5"("Array"=w63) -> ("Dynamic Data Type"=w83:dynamicdata)  [unwired: 3 in]
    n43 = call "Convert to Dynamic Data3"("Array"=w63) -> ("Dynamic Data Type"=w86:dynamicdata)  [unwired: 3 in]
    n44 = call "Convert to Dynamic Data4"("Array"=w72) -> ("Dynamic Data Type"=w87:dynamicdata)  [unwired: 3 in]
    n45 = call "Convert to Dynamic Data7"("Array"=w63) -> ("Dynamic Data Type"=w80:dynamicdata)  [unwired: 3 in]
    n46 = call "Convert to Dynamic Data8"("Array"=w70) -> ("Dynamic Data Type"=w81:dynamicdata)  [unwired: 3 in]
    n47 = call "Build XY Graph"("Y Input"=w113, "X Input"=w112) -> ("XY Graph"=→"I vs Chan 0":cluster{"X":dbl[], "Y":dbl[]}[])  [unwired: 8 in, 1 out]
    n48 = call "Build XY Graph3"("Y Input"=w84, "X Input"=w83) -> ("XY Graph"=→"I vs Chan 2":cluster{"X":dbl[], "Y":dbl[]}[])  [unwired: 8 in, 1 out]
    n49 = call "Build XY Graph2"("Y Input"=w87, "X Input"=w86) -> ("XY Graph"=→"I vs Chan 1":cluster{"X":dbl[], "Y":dbl[]}[])  [unwired: 8 in, 1 out]
    n50 = call "Build XY Graph4"("Y Input"=w81, "X Input"=w80) -> ("XY Graph"=→"I vs Chan 3":cluster{"X":dbl[], "Y":dbl[]}[])  [unwired: 8 in, 1 out]
    n51 = case shown="True" w99 {
      tunnel: w93 -> [w163 w168]
      tunnel: [w163 w168] -> w96
      tunnel: w92 -> [w164 w167]
      tunnel: w68 -> [_ w166]
      tunnel: [w164 w165] -> w91
      frame False {
      }
      frame True {
        n52 = Insert Into Array(array=w167, new element=w166) -> (w165:dbl[])  [unwired: 1 in]
      }
    }
    n53 = case shown="True" w98 {
      tunnel: w96 -> [w157 w162]
      tunnel: [w157 w162] -> w95
      tunnel: w91 -> [w158 w161]
      tunnel: w67 -> [_ w160]
      tunnel: [w158 w159] -> w90
      frame False {
      }
      frame True {
        n54 = Insert Into Array(array=w161, new element=w160) -> (w159:dbl[])  [unwired: 1 in]
      }
    }
    n55 = case shown="True" w97 {
      tunnel: w95 -> [w151 w153]
      tunnel: w90 -> [w152 w156]
      tunnel: w66 -> [_ w155]
      tunnel: [w152 w154] -> w89
      tunnel: [w151 w153] -> w88
      frame False {
      }
      frame True {
        n56 = Insert Into Array(array=w156, new element=w155) -> (w154:dbl[])  [unwired: 1 in]
      }
    }
    n57 = call-poly <vilib>:"Write Delimited Spreadsheet.vi"("file path (dialog if empty)"=w117, "format (%.3f)"="%.9e", "1D data"=w89, "append to file? (new file:F)"=TRUE, "error in (no error)"=w88, "transpose? (no:F)"=FALSE, "delimiter (\\t)"="\t" ("delimiter (\\t)")) -> ("error out"=w78:errorcluster)  [unwired: 7 in, 1 out]
  }
  n58 = call "Stop cRIO DAQ.vi"("DAQ_AI_Reader endpoint"=w17, "DAQ_CMD_Writer endpoint"=w18, "error in (no error)"=w10, "VI reference"=w31, "application reference"=w32) -> ("error out"=→"error out":errorcluster)  [unwired: 6 in]
  "Name 0" <- "Channel name 0"
  "Name 1" <- "Channel name 1"
  "Name 2" <- "Channel name 2"
  "Name 3" <- "Channel name 3"
